vi "LoadPauseProgram.vi"(8 "error in (no error)":errorcluster, 11 "Motion Settings":T1 {"3rd Axis" items=["x", "y", "z", "w"]; "Xtra planes" min=1; "Xtra plane\ndistance  (um)" min=0; "Distance between\nscan planes (um)" format="%.2f"; "Distance between\nscan lines (um)" format="%.2f"; "SMAC Axis" items=["None"=0, "Axis 1"=1, "Axis 2"=2, "Axis 3"=3, "Axis 4"=4, "Axis 5"=5, "Axis 6"=6, "Axis 7"=7, "Axis 8"=8, "Vector Space 1"=17, "Vector Space 2"=18, "Vector Space 3"=19, "Vector Space 4"=20]; "Motion Bd ID" min=1 max=32 step=1}) -> (0 "error out":errorcluster)   [LabVIEW 2022 SP3]
uses:
  MotionParameters.ctl
  MotionSys.ctl
  -MotionRoutines/ScanAxis.ctl
  -MotionRoutines/3rdAxis.ctl
  <vilib>/Motion/FlexMotion/FunctionsVIs/OnboardProgramming.llb/Pause/Resume Program.flx
  <vilib>/Motion/FlexMotion/CustomControls/CustomControls.llb/Program.flx
  <vilib>/Motion/FlexMotion/CustomControls/CustomControls.llb/Resource Out.flx
panel:
  # "1-D and 2-D B scan settings"
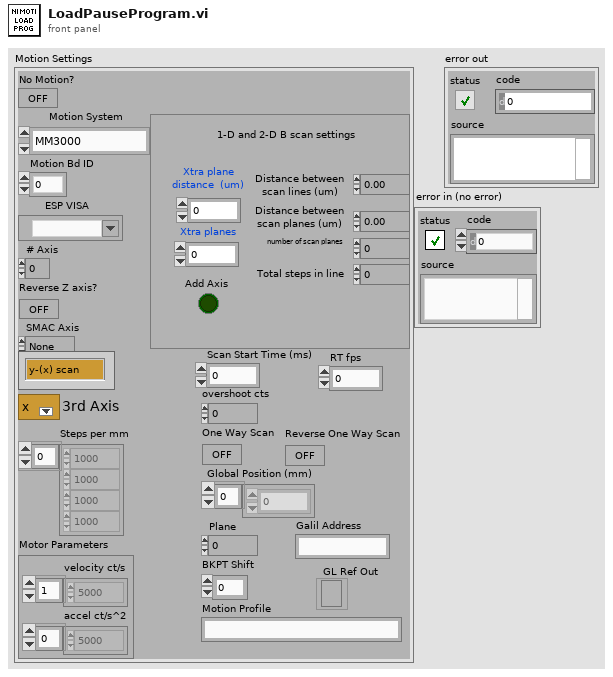
[diagram p1: front panel]
types:
  T1 = typedef "MotionParameters.ctl" = cluster{"No Motion?":bool, "Motion System":T2, "Motion Bd ID":u8, "Motion Profile":string, "# Axis":i8, "Reverse Z axis?":bool, "SMAC Axis":u16, "scan pair":T3, "RT fps":sgl, "Steps per mm":i32[], "Motor Parameters":cluster{"velocity ct/s":dbl[], "accel ct/s^2":dbl[]}, "One Way Scan":bool, "Reverse One Way Scan":bool, "Global Position (mm)":dbl[], "Plane":i32, "Distance between\nscan lines (um)":sgl, "Distance between\nscan planes (um)":sgl, "number of scan planes":i32, "Total steps in line":i32, "Xtra plane\ndistance  (um)":i32, "Xtra planes ":i32, "Add Axis":bool, "overshoot cts":i32, "BKPT Shift":i32, "Scan Start Time (ms)":u32, "ESP VISA":refnum<visa-resource-name>, "3rd Axis":T4, "GL Ref Out":refnum<k7>, "Galil Address":string}
  T2 = typedef "MotionSys.ctl" = enum16{"MM3000", "NI 735x", "Newport ESP", "No Motion Card", "Galil"}
  T3 = typedef "ScanAxis.ctl" = enum16{"y-(x) scan", "x-(y) scan", "z-(x) scan", "z-(y) scan", "y-(z) scan", "x-(z) scan", "w-(x) scan", "w-(y) scan", "w-(z) scan", "x-(w) scan", "y-(w) scan", "z-(w) scan"}
  T4 = typedef "3rdAxis.ctl" = u16
  T5 = typedef "Resource Out.flx" = u8
  T6 = typedef "Program.flx" = u8
  T7 = typedef "Bd Id Out" = u8
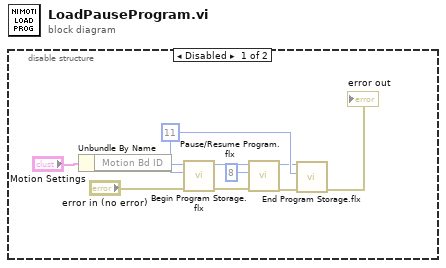
[diagram p0: block diagram]
diagram:
  n1 = disable-structure shown="Disabled" {
    frame Disabled {
      w6 = T6 11 ("Program (1)")
      n2 = Unbundle By Name("Motion Settings") -> ("Motion Bd ID"=w10:u8)
      n3 = call <vilib>:"Begin Program Storage.flx"("error in (no error)"="error in (no error)", "Program (1)"=w6, "Board ID"=w10) -> ("error out"=w3:errorcluster, "Bd ID Out"=w2:T7)  [unwired: 3 in, 1 out]
      n4 = call "Pause/Resume Program.flx"("error in (no error)"=w3, "Program (1)"=T5 8 ("Resource Out"), "Board ID"=w2) -> ("error out"=w5:errorcluster, "Bd ID Out"=w4:T7)  [unwired: 3 in, 1 out]
      n5 = call <vilib>:"End Program Storage.flx"("error in (no error)"=w5, "Program (1)"=w6, "Board ID"=w4) -> ("error out"=→"error out":errorcluster)  [unwired: 3 in, 2 out]
    }
    frame Enabled {
    }
  }
